vi "Configure System Channels.vi"(0 "VISA resource name":refnum<visa-resource-name>, 1 "Unit Address (1)":i16=1, 2 "Input Fail (0.0)":dbl format="%.2f", 3 "Open Loop Channel (F: Off)":bool, 5 "Channel (1)":i16=1, 7 "Guarantee Soak Band (1.0)":dbl=1.0 format="%.2f", 9 "Channel Autotune Set Point (90.0)":dbl=90.0 format="%.2f", 11 "error in (no error)":errorcluster {"code" format="%.0x"}) -> (4 "VISA resource name out":refnum<visa-resource-name>, 15 "error out":errorcluster {"code" format="%.0x"})   [LabVIEW 2010]
doc: "This VI defines the global operating characteristics of the controller channels."
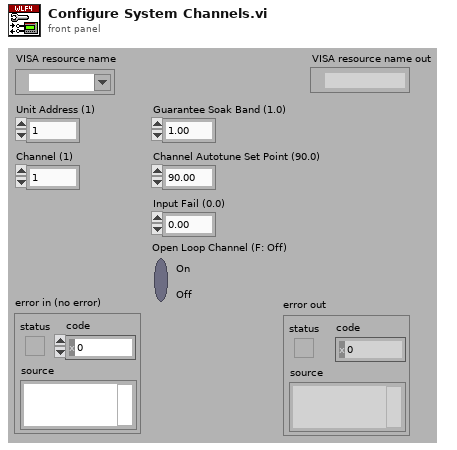
[diagram p1: front panel]
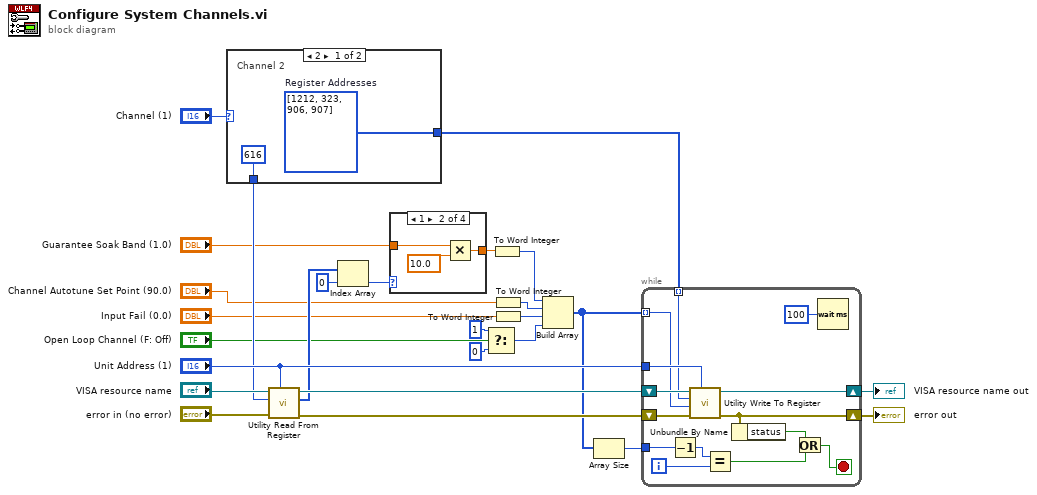
[diagram p0: block diagram]
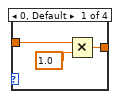
[diagram p2: hidden frame]
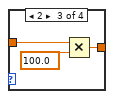
[diagram p3: hidden frame]
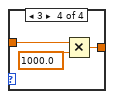
[diagram p4: hidden frame]
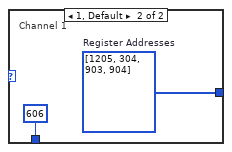
[diagram p5: hidden frame]
diagram:
  n1 = case shown="2" "Channel (1)" {
    tunnel: [616 606] -> w18
    tunnel: [w27 w29] -> w9
    frame 2 {
      w27 = i32[] [1212, 323, 906, 907]  # Register Addresses
      # "Channel 2"
    }
    frame 1, Default {
      w29 = i32[] [1205, 304, 903, 904]  # Register Addresses
      # "Channel 1"
    }
  }
  n2 = call "Utility Read From Register.vi"("Unit Address (1)"="Unit Address (1)", "error in (no error)"="error in (no error)", "Register Address (0)"=w18, "VISA resource name"="VISA resource name") -> ("error out"=w19:errorcluster, "Data"=w16:i16[], "VISA resource name out"=w20:refnum<visa-resource-name>)  [unwired: 5 in]
  n3 = Index Array(array=w16, index=0) -> (element=w15:i16)
  n4 = case shown="1" w15 {
    tunnel: "Guarantee Soak Band (1.0)" -> [w33 w36 w39 w42]
    tunnel: [w31 w34 w37 w40] -> w13
    frame 0, Default {
      n5 = Multiply(x=w33, y=1.0) -> (x*y=w31:dbl)
    }
    frame 1 {
      n6 = Multiply(x=w36, y=10.0) -> (x*y=w34:dbl)
    }
    frame 2 {
      n7 = Multiply(x=w39, y=100.0) -> (x*y=w37:dbl)
    }
    frame 3 {
      n8 = Multiply(x=w42, y=1000.0) -> (x*y=w40:dbl)
    }
  }
  n9 = Select(t=1, s="Open Loop Channel (F: Off)", f=0) -> (s? t:f=w3:i32)
  n10 = To Word Integer(number=w13) -> (16bit integer=w12:i16)
  n11 = To Word Integer(number="Channel Autotune Set Point (90.0)") -> (16bit integer=w7:i16)
  n12 = To Word Integer(number="Input Fail (0.0)") -> (16bit integer=w8:i16)
  n13 = Build Array(w12, w7, w8, w3) -> (w11:i32[])
  n14 = Array Size(array=w11) -> (size(s)=w10:i32)
  n15 = while {
    tunnel: "Unit Address (1)" -> [w56]
    shift-right: [w53] -> w26
    shift-left: w20 -> [w55]
    shift-right: [w51] -> w25
    shift-left: w19 -> [w54]
    tunnel: w11 -> [w50] mode=indexing
    tunnel: w10 -> [w44]
    tunnel: w9 -> [w43] mode=indexing
    i -> [w49]
    stop <- w48 stop-if-true
    n16 = Decrement(x=w44) -> (x-1=w45:i32)
    n17 = call "Utility Write To Register.vi"("Unit Address (1)"=w56, "error in (no error)"=w54, "Data (0)"=w50, "Register Address (0)"=w43, "VISA resource name"=w55) -> ("error out"=w51:errorcluster, "VISA resource name out"=w53:refnum<visa-resource-name>)  [unwired: 5 in]
    n18 = Equal?(x=w45, y=w49) -> (x = y?=w47:bool)
    n19 = Unbundle By Name(w51) -> ("status"=w46:bool)
    n20 = Or(x=w46, y=w47) -> (x .or. y?=w48:bool)
    n21 = Wait (ms)(milliseconds to wait=u32 100) -> ()  [unwired: 1 out]
  }
  "error out" <- w25
  "VISA resource name out" <- w26
